vi "Main.vi"() -> ()   [LabVIEW 2024]
uses:
  <vilib>/Instr/_visa.llb/VISA Configure Serial Port (Instr).vi
panel:
  out "Waveform Graph":dynamicdata(graph)
  in  "Fault Injection":bool
  out "State":enum16{"IDLE", "START", "RUN", "STOP"}(ring)
  in  "CONTROLS":T1 {"Phase Data" min=0.0 max=360.0 step=0.08789; "Frequency Data (Hz)" min=0.0 max=37500000.0 step=1.0 format="%#_10g"}
  out "error out":errorcluster
  out "VISA resource name out":refnum<visa-resource-name>
  out "RX":string
  out "TX":string
  in  "VISA resource name":refnum<visa-resource-name>="com3" caption="Boud rate: 115200"
  out "CRC":bool
  in  "Send Button":bool
  out "INDICATORS":T1 {"Frequency Data (Hz)" format="%#_9g"}
  out "NACK":bool
  out "ACK":bool
  in  "Close Button":bool
  in  "stop":bool
  in  "Start Button":bool
  # "SIGNAL GENERATOR GUI | 1V000"
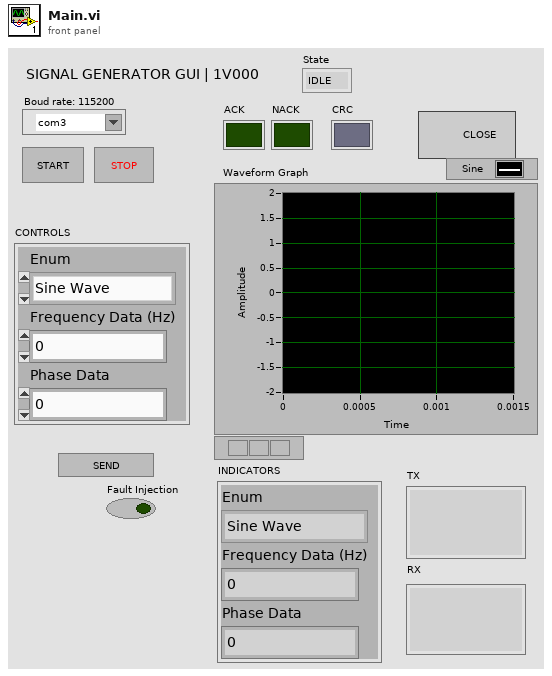
[diagram p1: front panel]
types:
  T1 = cluster{"Enum":enum16{"Sine Wave", "Triangular Wave", "Square Wave"}, "Frequency Data (Hz)":dbl, "Phase Data":dbl}
  T2 = enum16{"Sine Wave", "Triangular Wave", "Square Wave"}
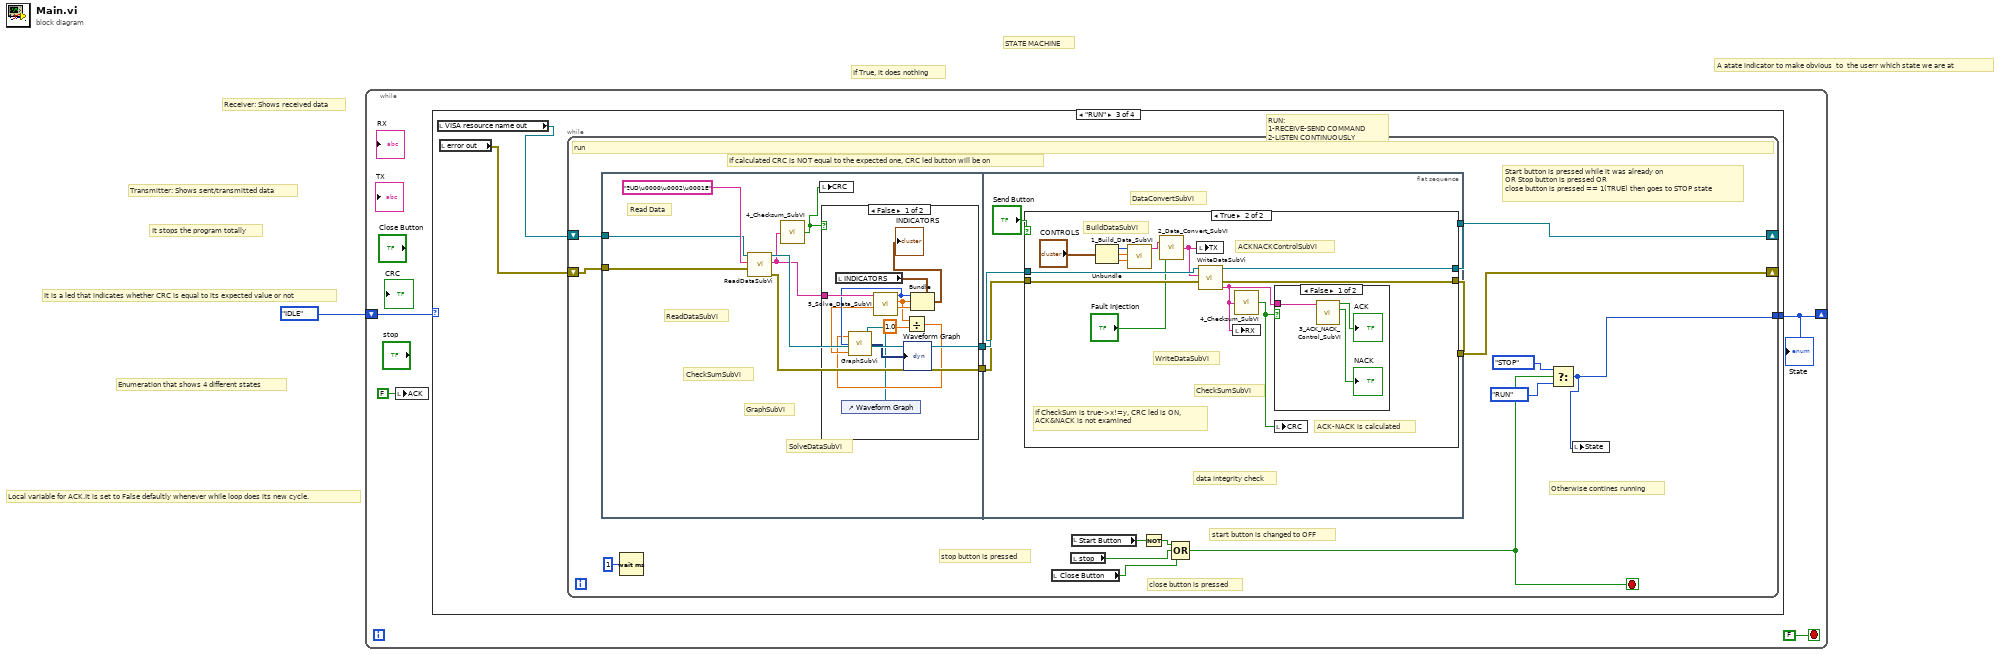
[diagram p0: block diagram]
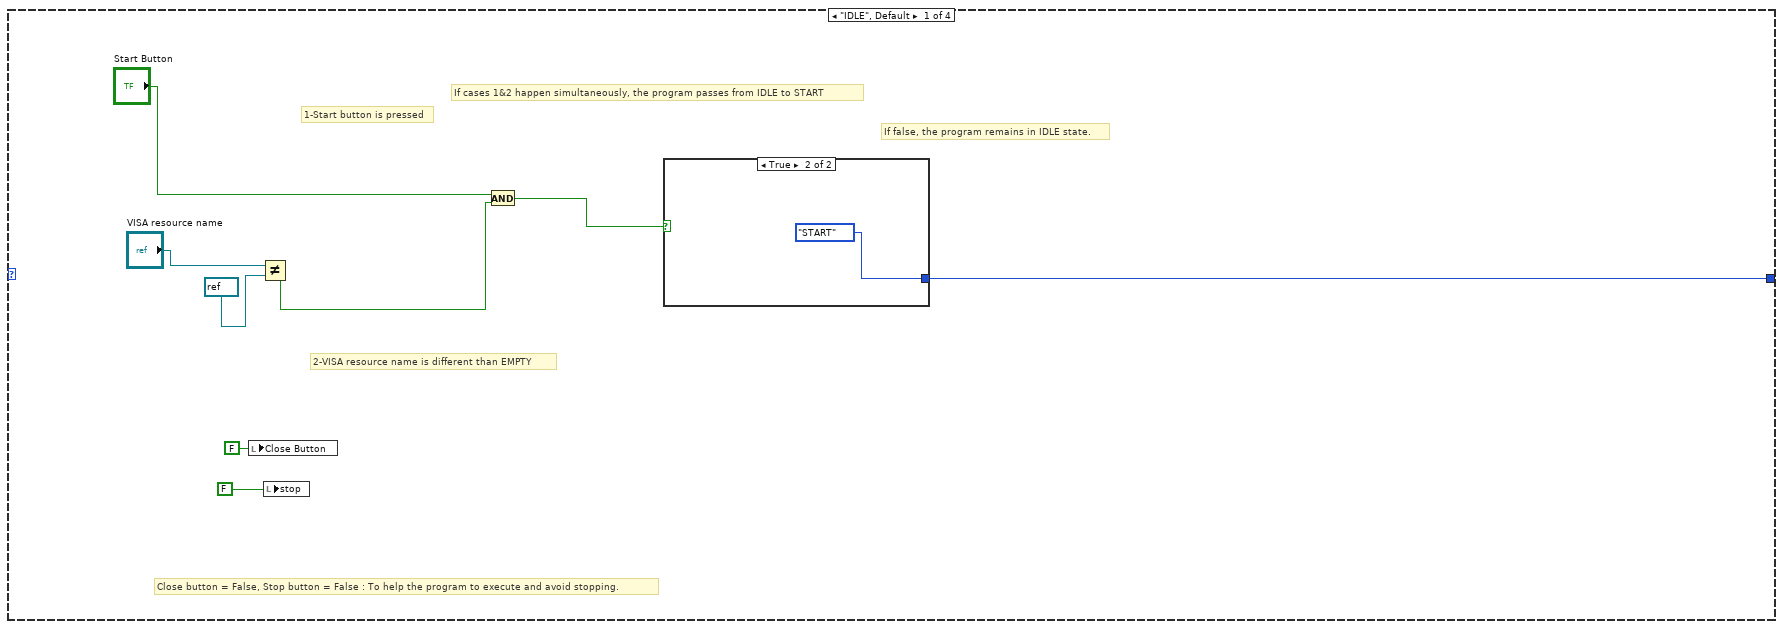
[diagram p2: hidden frame]
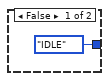
[diagram p3: hidden frame]
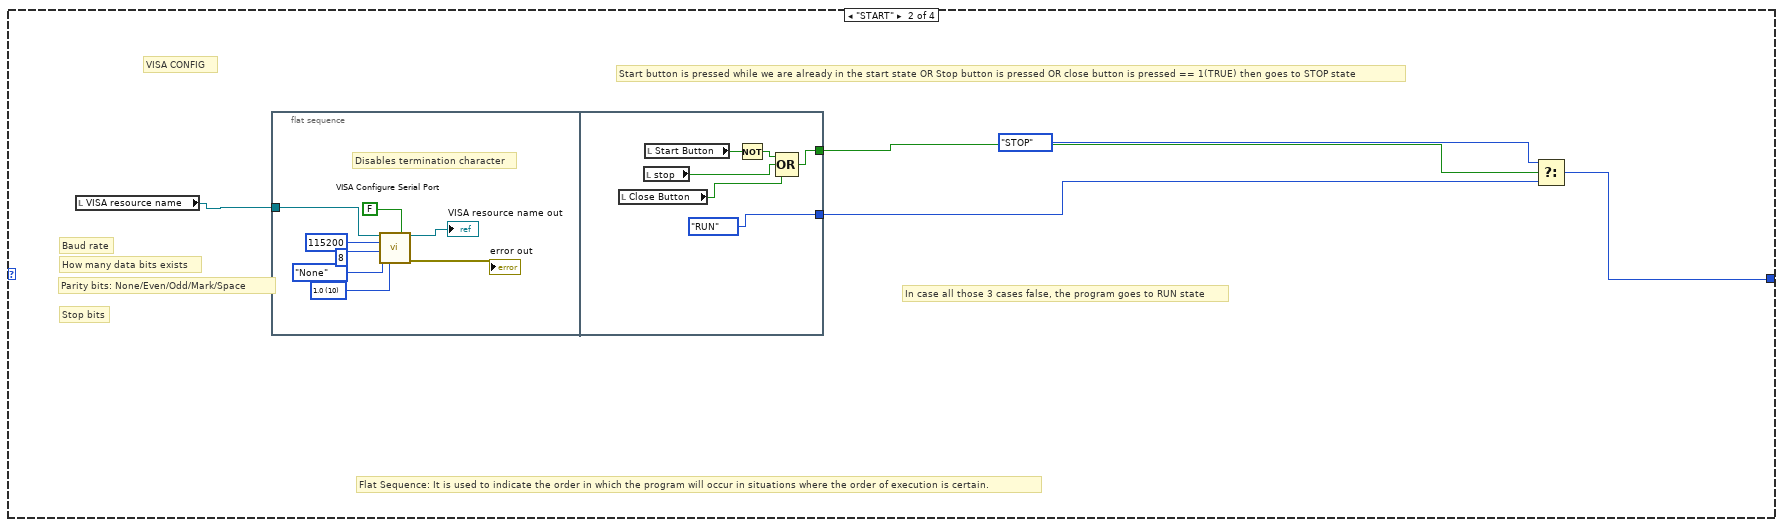
[diagram p4: hidden frame]
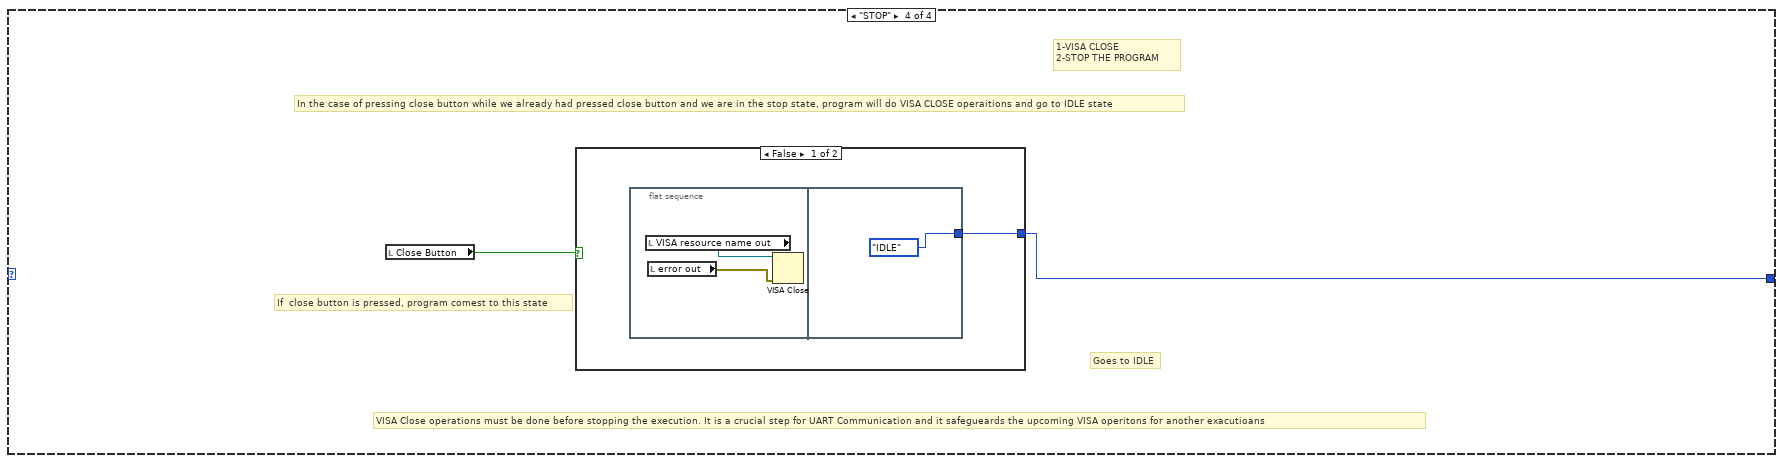
[diagram p8: hidden frame]
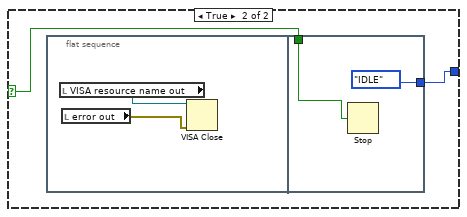
[diagram p9: hidden frame]
diagram:
  # "If True, it does nothing"
  # "STATE MACHINE"
  # "Local variable for ACK.It is set to False defaultly whenever while loop does its new cycle."
  # "It is a led that indicates whether CRC is equal to its expected value or not"
  # "It stops the program totally"
  # "Transmitter: Shows sent/transmitted data"
  # "Receiver: Shows received data"
  # "Enumeration that shows 4 different states"
  # "A atate indicator to make obvious  to  the userr which state we are at"
  n1 = while {
    shift-right: [w3] -> _
    shift-left: enum16{"IDLE", "START", "RUN", "STOP"}."IDLE" -> [w4]
    stop <- FALSE stop-if-true
    n2 = local write "ACK"(FALSE ("ACK")) -> ()
    n3 = case shown="\"RUN\"" w4 {
      tunnel: [w9 w19 w35 w93] -> w3
      frame "IDLE", Default {
        # "If false, the program remains in IDLE state."
        # "If cases 1&2 happen simultaneously, the program passes from IDLE to START"
        # "Close button = False, Stop button = False : To help the program to execute and avoid stopping."
        # "2-VISA resource name is different than EMPTY"
        # "1-Start button is pressed"
        n4 = local write "Close Button"(FALSE ("Close Button")) -> ()
        n5 = Not Equal?(x="VISA resource name", y=refnum<visa-resource-name> refnum) -> (x != y?=w11:bool)
        n6 = local write "stop"(FALSE ("Close Button")) -> ()
        n7 = And(x="Start Button", y=w11) -> (x .and. y?=w8:bool)
        n8 = case shown="True" w8 {
          tunnel: [enum16{"IDLE", "START", "RUN", "STOP"}."IDLE" enum16{"IDLE", "START", "RUN", "STOP"}."START"] -> w9
          frame False {
          }
          frame True {
          }
        }
      }
      frame "START" {
        # "In case all those 3 cases false, the program goes to RUN state"
        # "Start button is pressed while we are already in the start state OR Stop button is pressed OR close button is pressed == 1(TRUE) then goes to STOP state"
        # "Baud rate"
        # "Stop bits"
        # "Parity bits: None/Even/Odd/Mark/Space"
        # "How many data bits exists"
        # "VISA CONFIG"
        # "Flat Sequence: It is used to indicate the order in which the program will occur in situations where the order of execution is certain."
        n9 = local read "VISA resource name"() -> (w18:refnum<visa-resource-name>)
        n10 = flat-sequence {
          tunnel: w18 -> [w23]
          tunnel: [w29] -> w17
          tunnel: [enum16{"IDLE", "START", "RUN", "STOP"}."RUN"] -> w16
          frame #0 {
            w25 = u16 10 items=["1.0"=10, "1.5"=15, "2.0"=20] ("stop bits (10: 1 bit)")
            # "Disables termination character"
            n11 = call-poly "VISA Configure Serial Port"("VISA resource name"=w23, "Enable Termination\nChar (T)"=FALSE ("Enable Termination\nChar (T)"), "baud rate (9600)"=u32 115200, "data bits (8)"=u16 8, "parity (0:none)"=enum16{"None", "Odd", "Even", "Mark", "Space"}."None", "stop bits (10: 1 bit)"=w25) -> ("VISA resource name out"=→"VISA resource name out":refnum<visa-resource-name>, "error out"=→"error out":errorcluster)  [unwired: 8 in]
          }
          frame #1 {
            n12 = local read "Close Button"() -> (w30:bool)
            n13 = local read "stop"() -> (w31:bool)
            n14 = local read "Start Button"() -> (w34:bool)
            n15 = Not(x=w34) -> (.not. x?=w32:bool)
            n16 = Compound Arithmetic op=OR(w32, w31, w30) -> (w29:bool)
          }
        }
        n17 = Select(t=enum16{"IDLE", "START", "RUN", "STOP"}."STOP", s=w17, f=w16) -> (s? t:f=w19:enum16{"IDLE", "START", "RUN", "STOP"})
      }
      frame "RUN" {
        # "RUN:\n1-RECEIVE-SEND COMMAND\n2-LISTEN CONTINUOUSLY"
        n18 = local read "VISA resource name out"() -> (w37:refnum<visa-resource-name>)
        n19 = local read "error out"() -> (w36:errorcluster)
        n20 = while {
          shift-right: [w49] -> _
          shift-left: w37 -> [w47]
          shift-right: [w48] -> _
          shift-left: w36 -> [w46]
          tunnel: [w38] -> w35
          stop <- w39 stop-if-true
          # "close button is pressed"
          # "stop button is pressed"
          # "start button is changed to OFF"
          # "Otherwise contines running"
          # "Start button is pressed while it was already on\nOR Stop button is pressed OR \nclose button is pressed == 1(TRUE) then goes to STOP state"
          # "If calculated CRC is NOT equal to the expected one, CRC led button will be on"
          # "run"
          n21 = flat-sequence {
            tunnel: [w59] -> w52
            tunnel: [w57] -> w51
            tunnel: w47 -> [w54]
            tunnel: w46 -> [w53]
            tunnel: w52 -> [w73]
            tunnel: w51 -> [w72]
            tunnel: [w71] -> w49
            tunnel: [w70] -> w48
            frame #0 {
              # "GraphSubVi"
              # "SolveDataSubVi"
              # "Read Data"
              # "CheckSumSubVi"
              # "ReadDataSubVi"
              n22 = call "ReadDataSubVi.vi"("error in (no error)"=w53, "write buffer"="ªUD\u0000\u0002\u0001E", "VISA resource name"=w54) -> ("error out"=w57:errorcluster, "read buffer"=w55:string, "VISA resource name out"=w59:refnum<visa-resource-name>)  [unwired: 1 in, 1 out]
              n23 = call "4_Checksum_SubVI.vi"("data in"=w55) -> ("x != y?"=w56:bool)
              n24 = local write "CRC"(w56) -> ()
              n25 = case shown="False" w56 {
                tunnel: w55 -> [w69 _]
                frame False {
                  n26 = local read "INDICATORS"() -> (w68:T1)
                  n27 = control-ref of="Waveform Graph"() -> (w60:refnum<vi>)
                  n28 = call "5_Solve_Data_SubVI.vi"("String"=w69) -> ("Phase Data"=w65:dbl, "Frequency Data (Hz)"=w63:dbl, "Enum"=w66:T2)  [unwired: 8 in]
                  n29 = Divide(x=w63, y=1.0) -> (x/y=w61:dbl)
                  n30 = call "GraphSubVi.vi"("reference out"=w60, "Phase Data"=w65, "Waveform Type"=w66, "Frequency Data"=w61) -> ("Waveform Graph"=→"Waveform Graph":dynamicdata)  [unwired: 1 in]
                  n31 = Bundle(cluster=w68, "Enum"=w66, "Frequency Data (Hz)"=w63, "Phase Data"=w65) -> (→"INDICATORS":T1)
                }
                frame True {
                }
              }
            }
            frame #1 {
              # "data integrity check"
              # "DataConvertSubVi"
              n32 = case shown="True" "Send Button" {
                tunnel: w73 -> [w76 w84]
                tunnel: w72 -> [w75 w83]
                tunnel: [w76 w82] -> w71
                tunnel: [w75 w81] -> w70
                frame False {
                }
                frame True {
                  # "ACK-NACK is calculated"
                  # "If CheckSum is true->x!=y, CRC led is ON, \nACK&NACK is not examined"
                  # "CheckSumSubVi"
                  # "ACKNACKControlSubVi"
                  # "BuildDataSubVi"
                  # "WriteDataSubVi"
                  n33 = Unbundle("CONTROLS") -> ("Enum"=w88:T2, "Frequency Data (Hz)"=w87:dbl, "Phase Data"=w86:dbl)
                  n34 = call "1_Build_Data_SubVI.vi"("Phase Data"=w86, "Frequency Data"=w87, "Waveform Type"=w88) -> ("Message"=w85:string)  [unwired: 8 in]
                  n35 = call "2_Data_Convert_SubVI.vi"("hata sim"="Fault Injection", "data in"=w85) -> ("tx write"=w80:string)
                  n36 = local write "TX"(w80) -> ()
                  n37 = call "WriteDataSubVi.vi"("error in (no error)"=w83, "write buffer"=w80, "VISA resource name"=w84) -> ("read buffer"=w78:string, "error out"=w81:errorcluster, "VISA resource name out"=w82:refnum<visa-resource-name>)  [unwired: 1 in, 1 out]
                  n38 = local write "RX"(w78) -> ()
                  n39 = call "4_Checksum_SubVI.vi"("data in"=w78) -> ("x != y?"=w79:bool)
                  n40 = case shown="False" w79 {
                    tunnel: w78 -> [w92 _]
                    frame False {
                      n41 = call "3_ACK_NACK_Control_SubVI.vi"("String"=w92) -> ("NACK"=→"NACK":bool, "ACK"=→"ACK":bool)  [unwired: 9 in]
                    }
                    frame True {
                    }
                  }
                  n42 = local write "CRC"(w79) -> ()
                }
              }
            }
          }
          n43 = Wait (ms)(milliseconds to wait=u32 1) -> ()  [unwired: 1 out]
          n44 = local read "Close Button"() -> (w42:bool)
          n45 = local read "stop"() -> (w43:bool)
          n46 = local read "Start Button"() -> (w45:bool)
          n47 = Not(x=w45) -> (.not. x?=w44:bool)
          n48 = Compound Arithmetic op=OR(w44, w43, w42) -> (w39:bool)
          n49 = Select(t=enum16{"IDLE", "START", "RUN", "STOP"}."STOP", s=w39, f=enum16{"IDLE", "START", "RUN", "STOP"}."RUN") -> (s? t:f=w38:enum16{"IDLE", "START", "RUN", "STOP"})
          n50 = local write "State"(w38) -> ()
        }
      }
      frame "STOP" {
        # "In the case of pressing close button while we already had pressed close button and we are in the stop state, program will do VISA CLOSE operaitions and go to IDLE state"
        # "Goes to IDLE"
        # "1-VISA CLOSE\n2-STOP THE PROGRAM"
        # "VISA Close operations must be done before stopping the execution. It is a crucial step for UART Communication and it safegueards the upcoming VISA operitons for another exacutioans"
        # "If  close button is pressed, program comest to this state"
        n51 = local read "Close Button"() -> (w94:bool)
        n52 = case shown="False" w94 {
          selector: w94 -> [_ w100]
          tunnel: [w95 w99] -> w93
          frame False {
            n53 = flat-sequence {
              tunnel: [enum16{"IDLE", "START", "RUN", "STOP"}."IDLE"] -> w95
              frame #0 {
                n54 = local read "VISA resource name out"() -> (w97:refnum<visa-resource-name>)
                n55 = local read "error out"() -> (w96:errorcluster)
                n56 = VISA Close(VISA resource name=w97, error in (no error)=w96) -> ()  [unwired: 1 out]
              }
              frame #1 {
              }
            }
          }
          frame True {
            n57 = flat-sequence {
              tunnel: w100 -> [w104]
              tunnel: [enum16{"IDLE", "START", "RUN", "STOP"}."IDLE"] -> w99
              frame #0 {
                n58 = local read "VISA resource name out"() -> (w102:refnum<visa-resource-name>)
                n59 = local read "error out"() -> (w101:errorcluster)
                n60 = VISA Close(VISA resource name=w102, error in (no error)=w101) -> ()  [unwired: 1 out]
              }
              frame #1 {
                n61 = Stop(stop? (T)=w104) -> ()
              }
            }
          }
        }
      }
    }
    "State" <- w3
  }
